vi "Add TablePart.vi"(7 "Sheet Name":string, 8 "error in":errorcluster, 10 "TableDefinitionPart in":refnum<k24>, 11 "SpreadsheetDoc in":refnum<k24>) -> (0 "error out":errorcluster, 1 "TablePart":refnum<k24>, 2 "TableDefinitionPart out":refnum<k24>, 3 "SpreadsheetDoc out":refnum<k24>, 5 "Sheet Name":string)   [LabVIEW 2019, in "Open Xml.lvlib"]
uses:
  Open Xml.lvlib
  D:/git/Open-Xml-LabVIEW/Source/DocumentFormat.OpenXml.dll
  DocumentFormat.OpenXml.dll
  D:/git/Open-Xml-LabVIEW/Source/DocumentFormat.OpenXml.Framework.dll
  DocumentFormat.OpenXml.Framework.dll
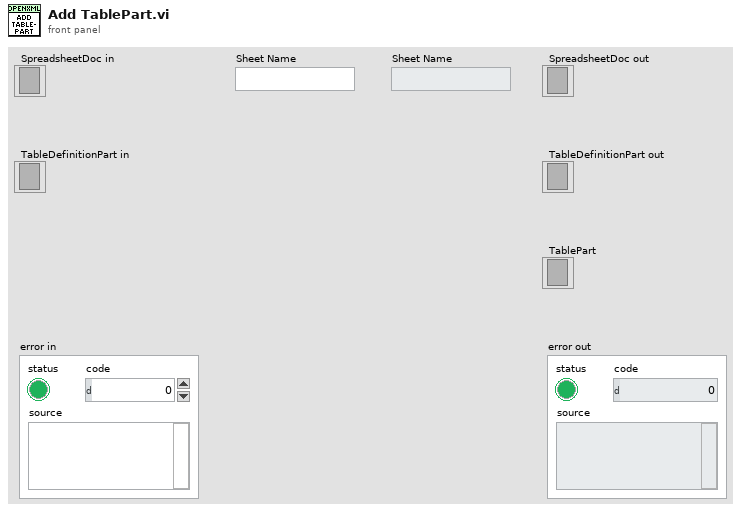
[diagram p1: front panel]
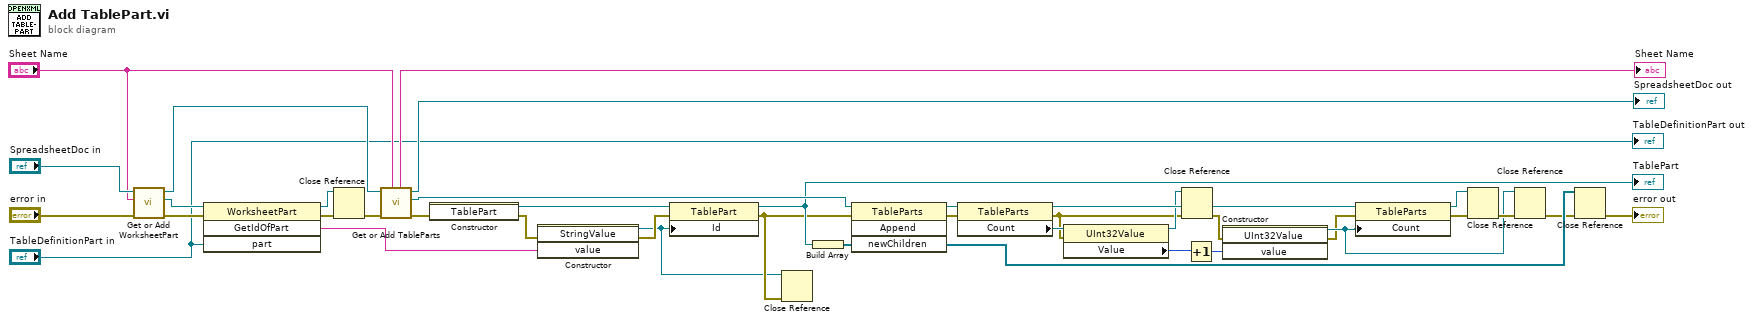
[diagram p0: block diagram]
diagram:
  n1 = call "Get or Add WorksheetPart.vi"("error in"="error in", "Sheet Name"="Sheet Name", "SpreadsheetDoc in"="SpreadsheetDoc in") -> ("error out"=w16:errorcluster, "WorksheetPart"=w11:refnum<k24>, "SpreadsheetDoc out"=w14:refnum<k24>)  [unwired: 6 in]
  n2 = invoke class="WorksheetPart" method="GetIdOfPart"(reference=w11, error in=w16, "part"="TableDefinitionPart in") -> (reference out=w6:refnum<k24>, error out=w12:errorcluster, "GetIdOfPart"=w10:string)  [unwired: 1 in, 1 out]
  n3 = Close Reference(reference=w6, error in (no error)=w12) -> (error out=w7:errorcluster)
  n4 = call "Get or Add TableParts.vi"("Sheet Name"="Sheet Name", "error in"=w7, "SpreadsheetDoc in"=w14) -> ("error out"=w32:errorcluster, "TableParts"=w34:refnum<k24>, "SpreadsheetDoc out"=→"SpreadsheetDoc out":refnum<k24>, "Sheet Name"=→"Sheet Name":string)  [unwired: 5 in]
  n5 = constructor class="TablePart"(error in=w32) -> (reference out=w18:refnum<k24>, error out=w9:errorcluster)  [unwired: 2 in, 1 out]
  n6 = constructor class="StringValue"(error in=w9, "value"=w10) -> (reference out=w4:refnum<k24>, error out=w8:errorcluster)  [unwired: 2 in, 2 out]
  n7 = property class="TablePart"(reference=w18, error in=w8, "Id"=w4) -> (reference out=w17:refnum<k24>, error out=w5:errorcluster)
  "TablePart" <- w17
  n8 = Close Reference(reference=w4, error in (no error)=w5) -> ()  [unwired: 1 out]
  n9 = Build Array(w17) -> (w38:refnum<k24>[])
  n10 = invoke class="TableParts" method="Append"(reference=w34, error in=w5, "newChildren"=w38) -> (reference out=w29:refnum<k24>, error out=w33:errorcluster, "newChildren"=w36:refnum<k24>[])  [unwired: 1 in, 1 out]
  n11 = property class="TableParts"(reference=w29, error in=w33) -> (reference out=w27:refnum<k24>, error out=w2:errorcluster, "Count"=w25:refnum<k24>)
  n12 = property class="UInt32Value"(reference=w25, error in=w2) -> (reference out=w22:refnum<k24>, "Value"=w24:u32)  [unwired: 1 out]
  n13 = Close Reference(reference=w22, error in (no error)=w2) -> (error out=w1:errorcluster)
  n14 = Increment(x=w24) -> (x+1=w23:u32)
  n15 = constructor class="UInt32Value"(error in=w1, "value"=w23) -> (reference out=w20:refnum<k24>, error out=w19:errorcluster)  [unwired: 2 in, 2 out]
  n16 = property class="TableParts"(reference=w27, error in=w19, "Count"=w20) -> (reference out=w26:refnum<k24>, error out=w28:errorcluster)
  n17 = Close Reference(reference=w26, error in (no error)=w28) -> (error out=w37:errorcluster)
  n18 = Close Reference(reference=w20, error in (no error)=w37) -> (error out=w21:errorcluster)
  n19 = Close Reference(reference=w36, error in (no error)=w21) -> (error out=→"error out":errorcluster)
  "TableDefinitionPart out" <- "TableDefinitionPart in"
